vi "AnalogOutput-Daemon.vi"(3 "Configuration":T2={"Output Lines"=["BNC_Panel/port0/line1", "BNC_Panel/port0/line2", "BNC_Panel/port0/line3"], "AO timestamp lines"=["BNC_Panel/port0/line0", "BNC_Panel/port0/line0", "BNC_Panel/port0/line0"]}, 4 "OutputRequest\nuser event refnum":T1) -> ()   [LabVIEW 2015]
doc: "OutputRequest handler for the AnalogOutput output device. \n\nThis VI is meant to be started asynchronously. It will register itself as a listener on the OutputRequest user event refnum and process any requests that it knows how to handle.\n\nThe \"Configuration\" structure is used for initialization and contains:\n\"Output Lines\": Array of device addresses for analog output\n\"AO timestamp lines\": Corresponding DO lines for timestamp\n\nCommands handled by this VI:\nTarget = \"all\"\n stop: Unregisters and stops running.\nTarget = \"analogOutput\"\n [index];sine;[freq]Hz;[amp]V;[length]ms;sample[freq]Hz;\n Produces a sine wave on the [index] output line. Also \n triggers a timestamp pulse if the configuration supports it."
uses:
  AnalogOutput-Configuration.ctl
  Typedefs/OutputRequest refnum.ctl
  Typedefs/OutputRequest.ctl
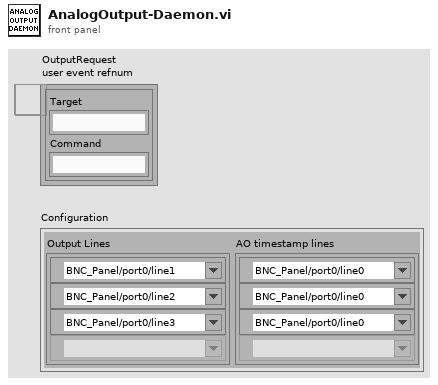
[diagram p1: front panel]
types:
  T1 = typedef "OutputRequest refnum.ctl" = refnum<user-event>
  T2 = typedef "AnalogOutput-Configuration.ctl" = cluster{"Output Lines":tag[], "AO timestamp lines":tag[]}
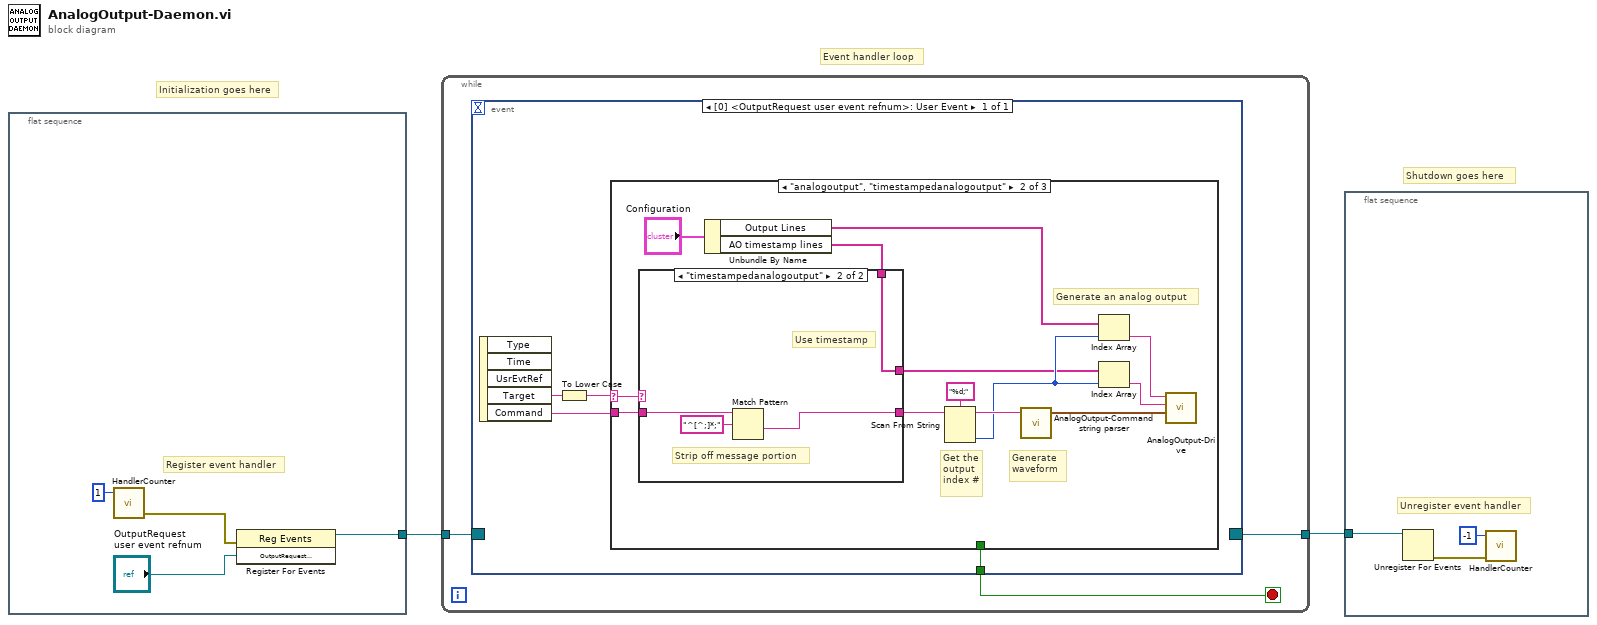
[diagram p0: block diagram]
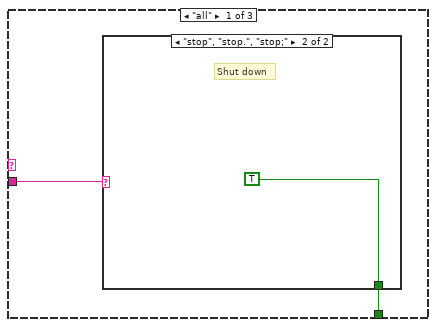
[diagram p2: hidden frame]
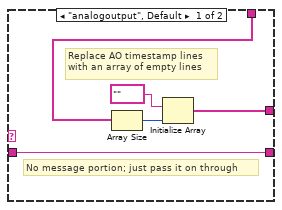
[diagram p4: hidden frame]
diagram:
  # "Shutdown goes here"
  # "Event handler loop"
  # "Initialization goes here"
  n1 = flat-sequence {
    tunnel: [w6] -> w2
    frame #0 {
      # "Register event handler"
      n2 = call "HandlerCounter.vi"("Change in count"=i16 1) -> ("error out"=w5:errorcluster)  [unwired: 3 in, 1 out]
      n3 = register-events(error in=w5, "OutputRequest\nuser event refnum") -> (reference out=w6:refnum<event-registration>)  [unwired: 1 in, 1 out]
    }
  }
  n4 = while {
    tunnel: w2 -> [w9]
    tunnel: [w8] -> w1
    stop <- w7 stop-if-true
    n5 = event shown="[0] <OutputRequest\nuser event refnum>: User Event" {
      selector: w9 -> [_]
      dyn-events: [_] -> w8
      timeout: _ -> [_]
      tunnel: [w13] -> w7
      event User Event {
        n6 = event-data() -> ("Target"=w12:string, "Command"=w10:string)  [unwired: 1 in, 3 out]
        n7 = To Lower Case(string=w12) -> (all lower case string=w11:string)
        n8 = case shown="\"analogoutput\", \"timestampedanalogoutput\"" w11 {
          selector: w11 -> [_ w21 _]
          tunnel: w10 -> [w15 w20 _]
          tunnel: [w14 _ _] -> w13
          frame "all" {
            n9 = case shown="\"stop\", \"stop.\", \"stop;\"" w15 {
              tunnel: [_ TRUE] -> w14
              frame Default {
                # "Unrecognized command.\nWe should probably put some\nerror throwing code here..."
              }
              frame "stop", "stop.", "stop;" {
                # "Shut down"
              }
            }
          }
          frame "analogoutput", "timestampedanalogoutput" {
            # "Generate\nwaveform"
            # "Get the\noutput\nindex #"
            # "Generate an analog output"
            n10 = Unbundle By Name("Configuration") -> ("Output Lines"=w25:tag[], "AO timestamp lines"=w19:tag[])
            n11 = case shown="\"timestampedanalogoutput\"" w21 {
              tunnel: w20 -> [w34 w37]
              tunnel: w19 -> [w30 w38]
              tunnel: [w32 w38] -> w18
              tunnel: [w34 w35] -> w17
              frame "analogoutput", Default {
                # "No message portion; just pass it on through"
                # "Replace AO timestamp lines\nwith an array of empty lines"
                n12 = Array Size(array=w30) -> (size(s)=w33:i32)
                n13 = Initialize Array(tag "" ("element"), w33) -> (w32:tag[])
              }
              frame "timestampedanalogoutput" {
                # "Strip off message portion"
                # "Use timestamp"
                n14 = Match Pattern(string=w37, regular expression="^[^;]*;") -> (after substring=w35:string)  [unwired: 1 in, 3 out]
              }
            }
            n15 = Scan From String(format string="%d;", input string=w17) -> (remaining string=w24:string, output 1=w22:i32)  [unwired: 3 in, 2 out]
            n16 = call "AnalogOutput-Command string parser.vi"("Command string"=w24) -> ("Waveform"=w29:waveform(dbl))  [unwired: 3 in, 1 out]
            n17 = Index Array(array=w25, index=w22) -> (element=w27:tag)
            n18 = Index Array(array=w18, index=w22) -> (element=w28:tag)
            n19 = call "AnalogOutput-Drive.vi"("Waveform"=w29, "Timestamp line"=w28, "Line"=w27) -> ()  [unwired: 8 in, 1 out]
          }
          frame Default {
            # "Ignore the request, it doesn't pertain\nto this output device"
          }
        }
      }
    }
  }
  n20 = flat-sequence {
    tunnel: w1 -> [w41]
    frame #0 {
      # "Unregister event handler"
      n21 = Unregister For Events(event registration refnum=w41) -> (error out=w40:errorcluster)  [unwired: 1 in]
      n22 = call "HandlerCounter.vi"("error in"=w40, "Change in count"=i16 -1) -> ()  [unwired: 2 in, 2 out]
    }
  }
